vi "GlobalLog.vi"() -> ()   [LabVIEW 2017]
panel:
  in  "PacketLog0Size":i32=100
  in  "PacketLog0Indx":i32
  out "PacketLog0":string[][](table)
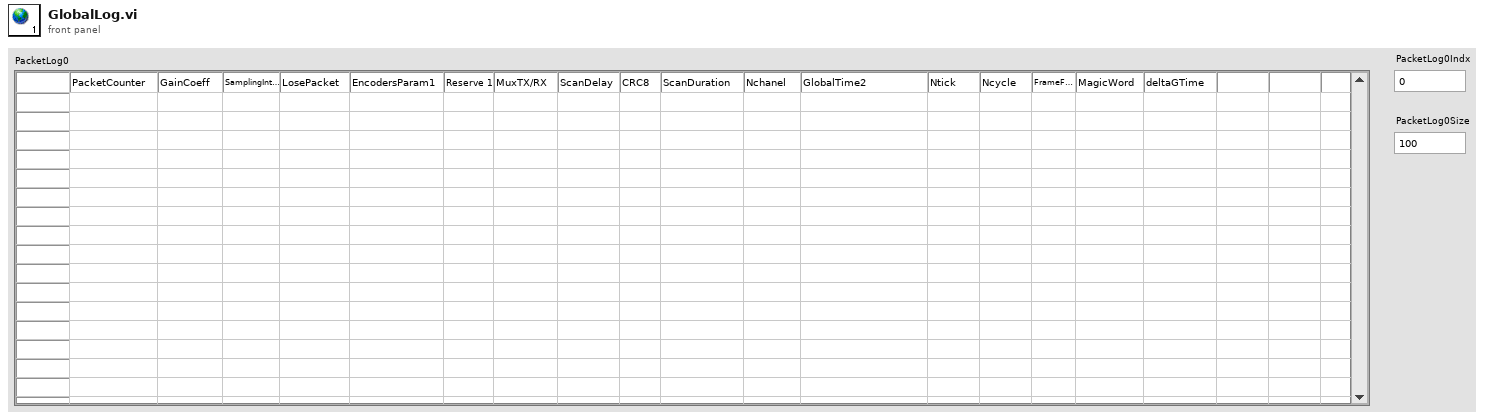
[diagram p1: front panel]
diagram:
